vi "Module DAQ teardown.vi"(8 "error in (no error)":errorcluster) -> (0 "error out":errorcluster)   [LabVIEW 2018]
doc: "_____\nCreated using Delacor QMH Event Scripter 5.0.0.112."
uses:
  Libraries/Module DAQ/Module DAQ.lvlib
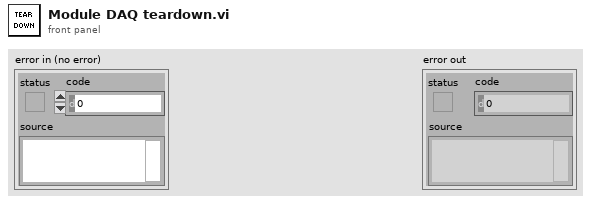
[diagram p1: front panel]
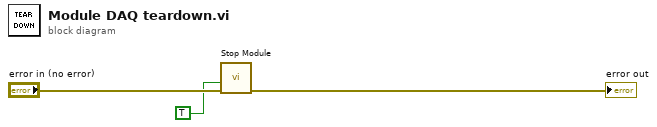
[diagram p0: block diagram]
diagram:
  n1 = call "Stop Module.vi"("error in (no error)"="error in (no error)", "Wait for Module to Stop? (F)"=TRUE) -> ("error out"=→"error out":errorcluster)  [unwired: 9 in]
